vi "Test Panel Retardation.vi"(8 "error in (no error)":errorcluster, 11 "VISA resource name":refnum<visa-resource-name>="COM4") -> (0 "error out":errorcluster, 3 "VISA resource name out":refnum<visa-resource-name>)   [LabVIEW 2017]
panel:
  out "Fraction of wave Retardation":dbl
  in  "Retardation":dbl=1.0 min=0.0 max=1.0 step=0.001
  in  "Numeric":i32
  in  "stop":bool
  out "query output":string
  out "read buffer 3":string
  in  "wavelength":dbl[unit] min=0.0 max=1.99999e-05 step=1.0000000000000002e-10
  out "Boolean":bool
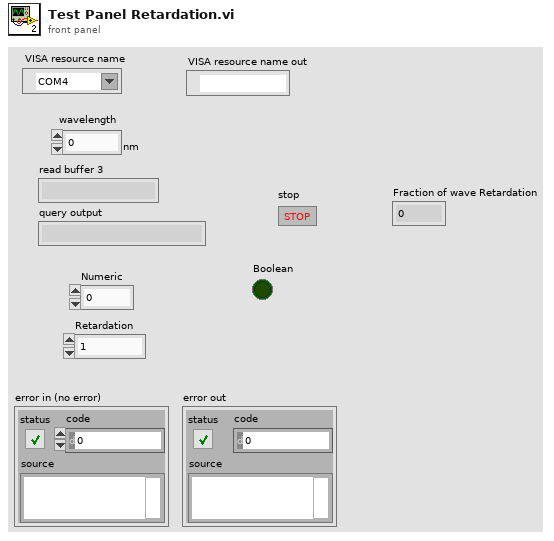
[diagram p1: front panel]
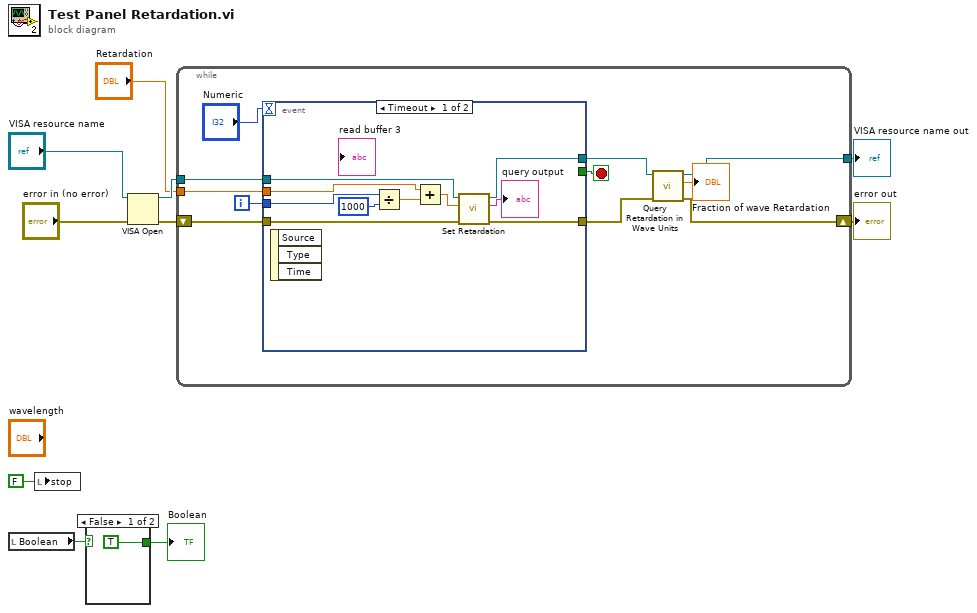
[diagram p0: block diagram]
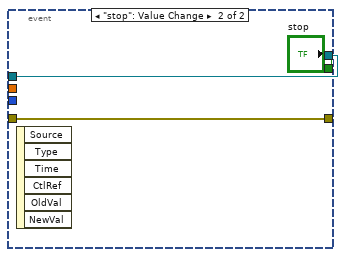
[diagram p2: hidden frame]
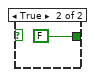
[diagram p3: hidden frame]
diagram:
  n1 = local read "Boolean"() -> (w8:bool)
  n2 = local write "stop"(FALSE ("stop")) -> ()
  n3 = case shown="False" w8 {
    tunnel: [TRUE FALSE] -> w7
    frame False {
    }
    frame True {
    }
  }
  "Boolean" <- w7
  n4 = VISA Open(error in (no error)="error in (no error)", VISA resource name="VISA resource name") -> (VISA resource name=w6:refnum<visa-resource-name>, error out=w5:errorcluster)  [unwired: 3 in]
  n5 = while {
    tunnel: w6 -> [w23]
    tunnel: [w14] -> w3
    tunnel: "Retardation" -> [w20]
    shift-right: [w16] -> w4
    shift-left: w5 -> [w22]
    i -> [w18]
    stop <- w21 stop-if-true
    n6 = event shown="[0] Timeout" {
      selector: _ -> [_ _]
      dyn-events: _ -> [_ _]
      timeout: "Numeric" -> [_ _]
      tunnel: w23 -> [w33 w35]
      tunnel: w22 -> [w32 w34]
      tunnel: [w30 w34] -> w17
      tunnel: [w29 w35] -> w15
      tunnel: [_ "stop"] -> w21
      tunnel: w20 -> [w28 _]
      tunnel: w18 -> [w24 _]
      event Timeout {
        n7 = event-data() -> ()  [unwired: 1 in, 3 out]
        n8 = Divide(x=w24, y=1000 ("x")) -> (x/y=w26:dbl)
        n9 = Add(x=w28, y=w26) -> (x+y=w27:dbl)
        n10 = call "Set Retardation.vi"("error in (no error)"=w32, "Retardation"=w27, "VISA resource name"=w33) -> ("error out"=w30:errorcluster, "query output"=→"query output":string, "VISA resource name out"=w29:refnum<visa-resource-name>)  [unwired: 6 in]
      }
      event "stop": Value Change {
        n11 = event-data() -> ()  [unwired: 1 in, 6 out]
      }
    }
    n12 = call "Query Retardation in Wave Units.vi"("error in (no error)"=w17, "VISA resource name"=w15) -> ("error out"=w16:errorcluster, "Fraction of wave Retardation"=→"Fraction of wave Retardation":dbl, "VISA resource name out"=w14:refnum<visa-resource-name>)  [unwired: 7 in]
  }
  "error out" <- w4
  "VISA resource name out" <- w3
